vi "Dispose.vi"(0 "reference in":refnum<class "G#Object.lvclass">, 5 "error in (no error)":errorcluster) -> (14 "reference out":refnum<class "G#Object.lvclass">, 19 "error out":errorcluster)   [LabVIEW 2020, in "G#Object.lvclass"]
doc: "Dispose all resources use by the object. This method will call dispose on all aggregated objects and then destroy them."
uses:
  <vilib>/addons/_AddQ/G#Object/G#Object.lvclass
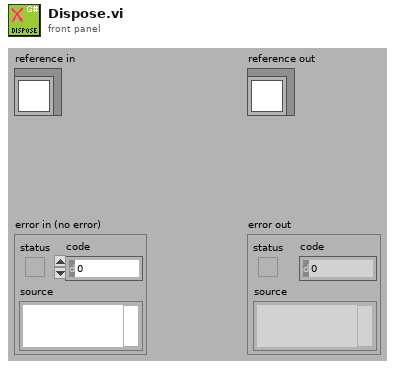
[diagram p1: front panel]
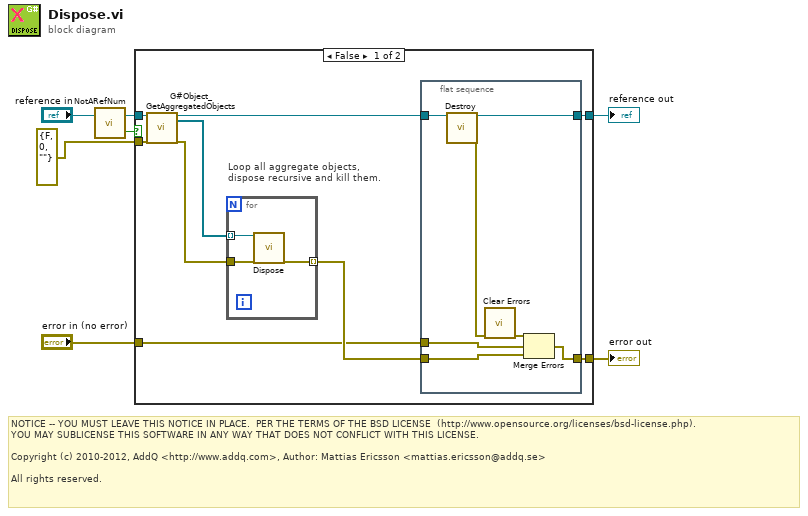
[diagram p0: block diagram]
diagram:
  # "NOTICE -- YOU MUST LEAVE THIS NOTICE IN PLACE.  PER THE TERMS OF THE BSD LICENSE  (http://www.opensource.org/licenses/bsd-license.php).\nYOU MAY SUBLICENSE THIS SOFTWARE IN ANY WAY THAT DOES NOT CONFLICT WITH THIS LICENSE.\n\nCopyright (c) 2010-2012, AddQ <http://www.addq.com>, Author: Mattias Ericsson <mattias.ericsson@addq.se>\n\nAll rights reserved."
  n1 = call-dynamic "NotARefNum.vi"("reference in"="reference in") -> ("not a refnum?"=w1:bool, "reference out"=w4:refnum<class "G#Object.lvclass">)  [unwired: 1 in]
  n2 = case shown="False" w1 {
    tunnel: errorcluster {"status"=FALSE, "code"=0, "source"=""} ("error in (no error)") -> [w14 _]
    tunnel: [w12 w27] -> w6
    tunnel: w4 -> [w11 w28]
    tunnel: [w9 w28] -> w3
    tunnel: "error in (no error)" -> [w8 w27]
    frame False {
      # "Loop all aggregate objects,\ndispose recursive and kill them."
      n3 = call <vilib>:"G#Object_GetAggregatedObjects.vi"("reference in"=w11, "error in (no error)"=w14) -> ("reference out"=w10:refnum<class "G#Object.lvclass">, "aggregated objects"=w15:refnum<class "G#Object.lvclass">[], "error out"=w16:errorcluster)  [unwired: 14 in, 1 out]
      n4 = for {
        tunnel: w15 -> [w25] mode=indexing
        tunnel: w16 -> [w26]
        tunnel: [w24] -> w13 mode=indexing
        n5 = call-dynamic "Dispose.vi"("reference in"=w25, "error in (no error)"=w26) -> ("error out"=w24:errorcluster)  [unwired: 16 in, 1 out]
      }
      n6 = flat-sequence {
        tunnel: w13 -> [w23]
        tunnel: [w22] -> w12
        tunnel: w10 -> [w21]
        tunnel: [w20] -> w9
        tunnel: w8 -> [w17]
        frame #0 {
          n7 = call-dynamic "Destroy.vi"("reference in"=w21) -> ("reference out"=w20:refnum<class "G#Object.lvclass">, "error out"=w19:errorcluster)  [unwired: 17 in]
          n8 = call <vilib>:"Clear Errors.vi"("error in (no error)"=w19) -> ("error out"=w18:errorcluster)  [unwired: 5 in, 1 out]
          n9 = Merge Errors(w18, w17, w23) -> (w22:errorcluster)
        }
      }
    }
    frame True {
    }
  }
  "error out" <- w6
  "reference out" <- w3
